vi "set_params.vi"(8 "error in (no error)":errorcluster, 11 "stresing in":refnum<class "stresing.lvclass">) -> (0 "error out":errorcluster, 3 "stresing out":refnum<class "stresing.lvclass">)   [LabVIEW 2019, in "stresing.lvlib" / "stresing.lvclass"]
uses:
  stresing.lvclass
  D:/github/TransientAbsorptionDAQ.lv/_camera/_camera.lvlibp/_cameraClass/_camera.lvclass
  stresing.lvclass/stresing.ctl
  _camera/_camera.lvlibp/_cameraClass/Read config file path.vi
  <vilib>/Utility/config.llb/Read Key (Path).vi
  <vilib>/Utility/config.llb/NI_LVConfig.lvlib
panel:
  in  "exposure":dbl=0.001 format="%.4f"
  in  "driver path":path=path "D:/driver/Stresing/ESLSCDLL/ESLSCDLL.dll"
  in  "OK Button":bool
  in  "number of blocks":u32=1
  in  "number of spectra":u32=2000
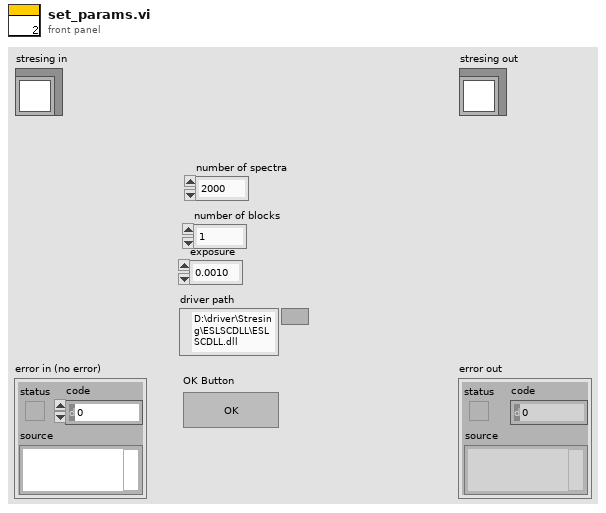
[diagram p1: front panel]
types:
  T1 = typedef "NI_LVConfig.lvlib/Config Data RefNum.ctl" = refnum<k1>
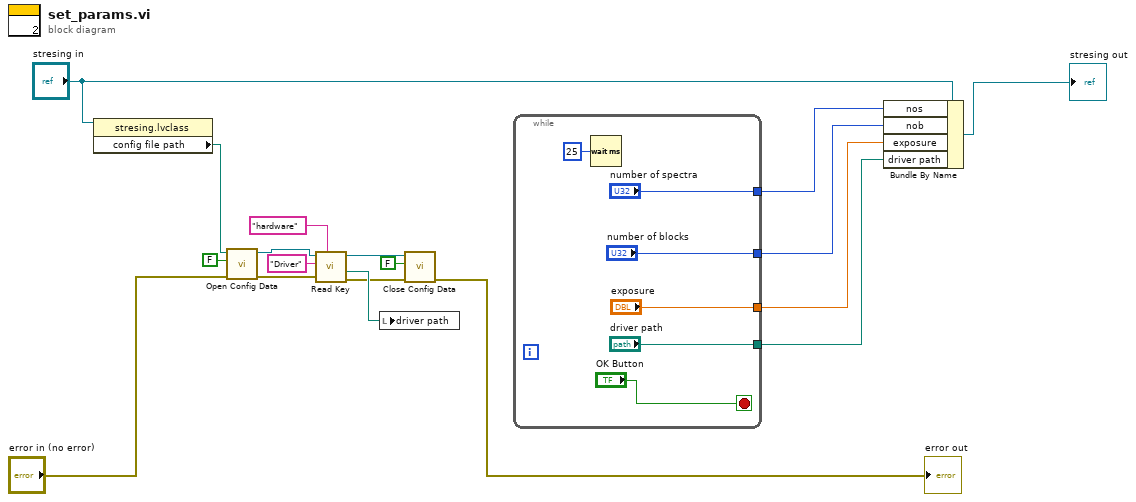
[diagram p0: block diagram]
diagram:
  n1 = property class="stresing.lvclass"(reference="stresing in") -> ("config file path"=w12:path)  [unwired: 1 in, 2 out]
  n2 = call <vilib>:"Open Config Data.vi"("error in (no error)"="error in (no error)", "create file if necessary (T)"=FALSE, "configuration file path"=w12) -> ("error out"=w3:errorcluster, "refnum"=w8:T1)  [unwired: 6 in, 1 out]
  n3 = call-poly <vilib>:"Read Key.vi"("section"="hardware", "error in (no error)"=w3, "key"="Driver", "refnum"=w8) -> ("error out"=w2:errorcluster, "value"=w7:path, "refnum out"=w5:T1)  [unwired: 4 in, 1 out]
  n4 = local write "driver path"(w7) -> ()
  n5 = call <vilib>:"Close Config Data.vi"("error in (no error)"=w2, "write file if changed (T)"=FALSE, "refnum"=w5) -> ("error out"=→"error out":errorcluster)  [unwired: 7 in, 1 out]
  n6 = while {
    tunnel: ["number of spectra"] -> w17
    tunnel: ["number of blocks"] -> w16
    tunnel: ["driver path"] -> w15
    tunnel: ["exposure"] -> w14
    stop <- "OK Button" stop-if-true
    n7 = Wait (ms)(milliseconds to wait=u32 25) -> ()  [unwired: 1 out]
  }
  n8 = Bundle By Name(cluster="stresing in", "nos"=w17, "nob"=w16, "exposure"=w14, "driver path"=w15) -> (→"stresing out":refnum<class "stresing.lvclass">)
